vi "PCE_format_ANSW.vi"(1 "Serial":bool, 2 "Réponse à envoyer":string) -> (0 "Chaine à envoyer":string)   [LabVIEW 2010]
panel:
  in  "Warning Code":u32
  in  "Error Code":u32
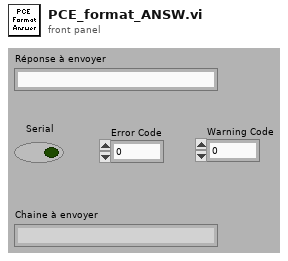
[diagram p1: front panel]
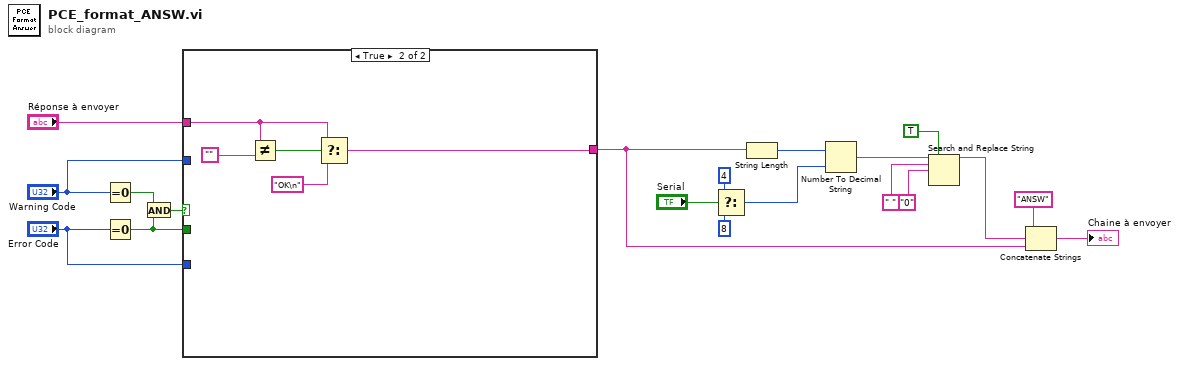
[diagram p0: block diagram]
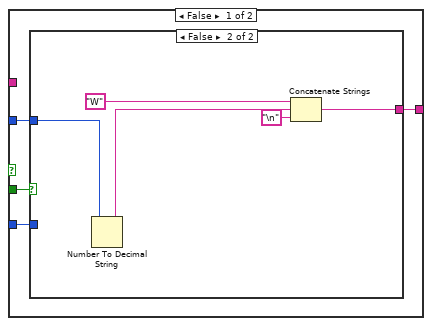
[diagram p2: hidden frame]
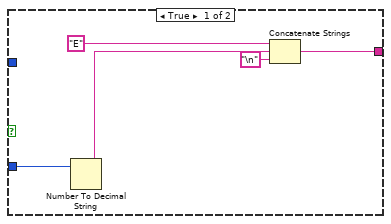
[diagram p3: hidden frame]
diagram:
  n1 = Equal To 0?(x="Warning Code") -> (x = 0?=w6:bool)
  n2 = Equal To 0?(x="Error Code") -> (x = 0?=w3:bool)
  n3 = And(x=w6, y=w3) -> (x .and. y?=w5:bool)
  n4 = case shown="True" w5 {
    tunnel: [w20 w34] -> w7
    tunnel: "Réponse à envoyer" -> [_ w36]
    tunnel: w3 -> [w23 _]
    tunnel: "Error Code" -> [w22 _]
    tunnel: "Warning Code" -> [w21 _]
    frame False {
      n5 = case shown="False" w23 {
        tunnel: w22 -> [w28 _]
        tunnel: w21 -> [_ w29]
        tunnel: [w27 w33] -> w20
        frame True {
          n6 = Number To Decimal String(number=w28) -> (decimal integer string=w26:string)  [unwired: 1 in]
          n7 = Concatenate Strings("E" ("string"), w26, "\n" ("string")) -> (w27:string)
        }
        frame False {
          n8 = Number To Decimal String(number=w29) -> (decimal integer string=w32:string)  [unwired: 1 in]
          n9 = Concatenate Strings("W" ("string"), w32, "\n" ("string")) -> (w33:string)
        }
      }
    }
    frame True {
      n10 = Not Equal?(x=w36, y="") -> (x != y?=w37:bool)
      n11 = Select(t=w36, s=w37, f="OK\n") -> (s? t:f=w34:string)
    }
  }
  n12 = Select(t=4, s="Serial", f=8) -> (s? t:f=w15:i32)
  n13 = String Length(string=w7) -> (length=w19:i32)
  n14 = Number To Decimal String(number=w19, width (-)=w15) -> (decimal integer string=w14:string)
  n15 = Search and Replace String(replace all?=TRUE ("replace all? (F)"), input string=w14, search string=" ", replace string="0" ("replace string (\"\")")) -> (result string=w10:string)  [unwired: 4 in, 3 out]
  n16 = Concatenate Strings("ANSW" ("string"), w10, w7) -> (→"Chaine à envoyer":string)
